vi "Open File.vi"(8 "error in":errorcluster, 11 "File Info":T1) -> (0 "error out":errorcluster)   [LabVIEW 2020, in "Peer Review.lvclass"]
uses:
  Peer Review.lvclass
  TypeDefs/File Info.ctl
  TypeDefs/File State.ctl
  TypeDefs/VI Type.ctl
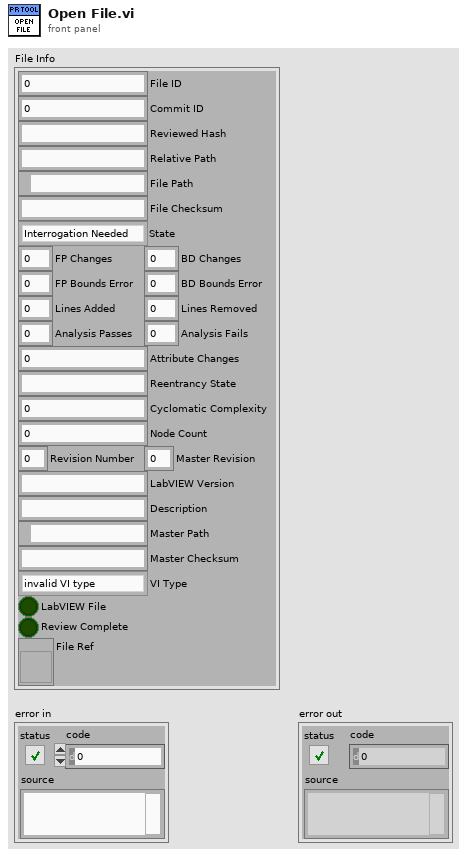
[diagram p1: front panel]
types:
  T1 = typedef "Peer Review.lvclass/File Info.ctl" = cluster{"File ID":i32, "Commit ID":i32, "Reviewed Hash":string, "Relative Path":string, "File Path":path, "File Checksum":string, "State":T2, "FP Changes":i32, "BD Changes":i32, "FP Bounds Error":dbl, "BD Bounds Error":dbl, "Lines Added":i32, "Lines Removed":i32, "Analysis Passes":i32, "Analysis Fails":i32, "Attribute Changes":i32, "Reentrancy State":string, "Cyclomatic Complexity":i32, "Node Count":i32, "Revision Number":u32, "LabVIEW Version":string, "Description":string, "Master Path":path, "Master Checksum":string, "VI Type":T3, "LabVIEW File":bool, "Review Complete":bool, "File Ref":refnum<vi>, "Master Revision":u32}
  T2 = typedef "Peer Review.lvclass/File State.ctl" = enum16{"Interrogation Needed", "Modified", "Deleted", "Added", "Matches Previous", "No Changes", "Moved", "Empty File"}
  T3 = typedef "Peer Review.lvclass/VI Type.ctl" = enum32{"invalid VI type", "Standard VI", "Control VI", "Global VI", "Polymorphic VI", "Configuration VI", "SubSystem", "Facade VI", "Method VI", "Statechart Diagram VI"}
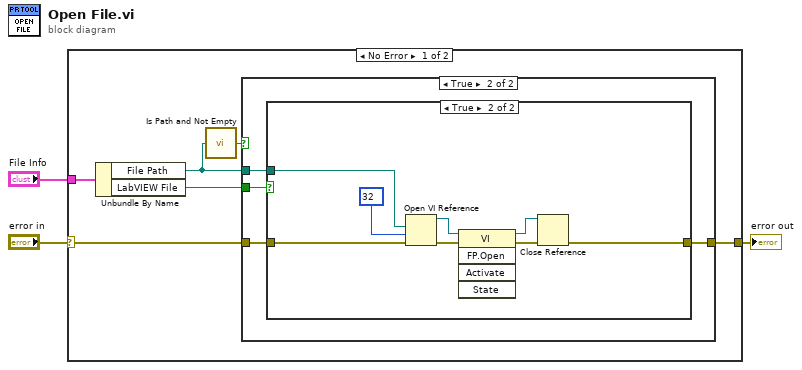
[diagram p0: block diagram]
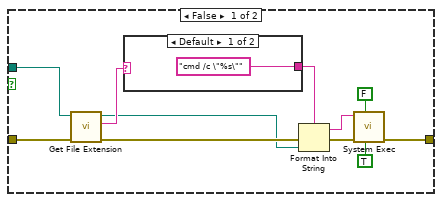
[diagram p3: hidden frame]
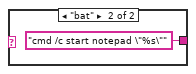
[diagram p4: hidden frame]
diagram:
  n1 = case shown="No Error" "error in" {
    selector: "error in" -> [w9 w36]
    tunnel: [w8 w36] -> w2
    tunnel: "File Info" -> [w7 _]
    frame No Error {
      n2 = Unbundle By Name(w7) -> ("File Path"=w5:path, "LabVIEW File"=w6:bool)
      n3 = call <vilib>:"Is Path and Not Empty.vi"("path"=w5) -> ("Is Path and Not Empty?"=w4:bool)  [unwired: 4 in]
      n4 = case shown="True" w4 {
        tunnel: w9 -> [w10 w14]
        tunnel: [w10 w13] -> w8
        tunnel: w6 -> [_ w12]
        tunnel: w5 -> [_ w11]
        frame False {
        }
        frame True {
          n5 = case shown="True" w12 {
            tunnel: w14 -> [w25 w35]
            tunnel: [w24 w30] -> w13
            tunnel: w11 -> [w15 w29]
            frame False {
              n6 = call <vilib>:"Get File Extension.vi"("error in (no error)"=w25, "file"=w15) -> ("error out"=w19:errorcluster, "lowercase file extension"=w17:string, "dup file"=w16:path)  [unwired: 5 in, 2 out]
              n7 = case shown="Default" w17 {
                tunnel: ["cmd /c \"%s\"" "cmd /c start notepad \"%s\""] -> w18
                frame Default {
                }
                frame "bat" {
                }
              }
              n8 = Format Into String(format string=w18, error in=w19, w16) -> (resulting string=w21:string, error out=w20:errorcluster)  [unwired: 1 in]
              n9 = call <vilib>:"System Exec.vi"("run minimized? (F)"=TRUE, "wait until completion? (T)"=FALSE, "error in (no error)"=w20, "command line"=w21) -> ("error out"=w24:errorcluster)  [unwired: 4 in, 3 out]
            }
            frame True {
              n10 = Open VI Reference(vi path=w29, options=32, error in (no error)=w35) -> (vi reference=w33:refnum<vi>, error out=w34:errorcluster)  [unwired: 3 in]
              n11 = invoke class="VI" method="FP.Open"(reference=w33, error in=w34) -> (reference out=w31:refnum<vi>, error out=w32:errorcluster)  [unwired: 3 in, 3 out]
              n12 = Close Reference(reference=w31, error in (no error)=w32) -> (error out=w30:errorcluster)
            }
          }
        }
      }
    }
    frame Error {
    }
  }
  "error out" <- w2
